vi "On Message.vi"(8 "error in (no error)":errorcluster, 10 "Actor in":refnum<class "Actor.lvclass">, 11 "Client Connection Handler Msg in":refnum<class "Client Connection Handler Msg.lvclass">) -> (0 "error out":errorcluster, 2 "Actor out":refnum<class "Actor.lvclass">, 3 "Client Connection Handler Msg out":refnum<class "Client Connection Handler Msg.lvclass">)   [LabVIEW 2021, in "Echo Broadcast Without Server Manager.lvlib" / "Client Connection Handler Msg.lvclass"]
uses:
  Client Connection Handler Msg.lvclass
  C:/Projects/WebSocket-Actor/WebSocket Actor/Abstract Messages/WebSocket Connection Handler Msg/WebSocket Connection Handler Msg.lvclass
  <vilib>/ActorFramework/Actor/Actor.lvclass
  WS Client/WS Client.lvclass
  C:/Program Files/National Instruments/LabVIEW 2021/vi.lib/ActorFramework/Actor/Actor.lvclass
  WebSocket Actor/Abstract Messages/WebSocket Connection Handler Msg/WebSocket Connection Handler Msg.lvclass/WebSocket Connection Handler Msg.ctl
  WebSocket Actor/Abstract Messages/WebSocket Connection Handler Msg/properties/Read Data.vi
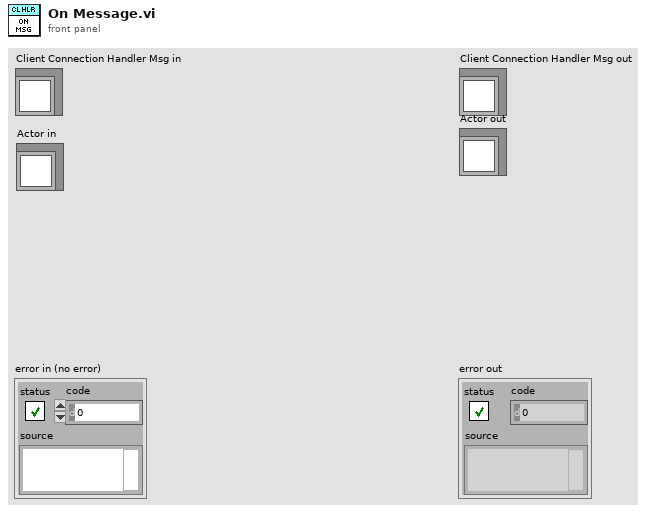
[diagram p1: front panel]
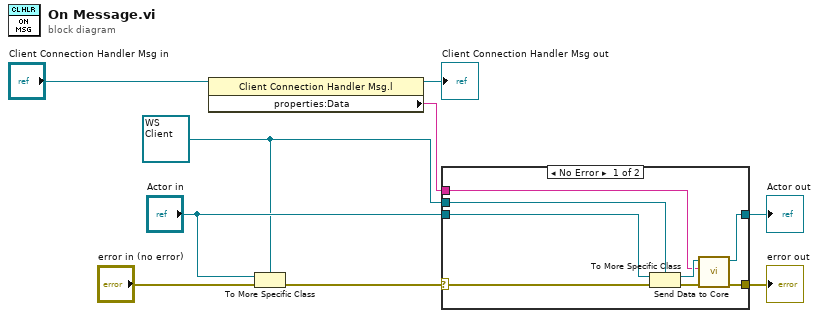
[diagram p0: block diagram]
diagram:
  w3 = refnum<class "WS Client.lvclass"> refnum ("WS Full LabVIEW Test.lvlib:WS Test Client.lvclass")
  n1 = property class="Client Connection Handler Msg.l"(reference="Client Connection Handler Msg in") -> (reference out=→"Client Connection Handler Msg out":refnum<class "Client Connection Handler Msg.lvclass">, "properties:Data"=w2:string)  [unwired: 1 in, 1 out]
  n2 = To More Specific Class(target class=w3, reference="Actor in", error in="error in (no error)") -> (error out=w9:errorcluster)  [unwired: 1 out]
  n3 = case shown="No Error" w9 {
    selector: w9 -> [w16 w18]
    tunnel: "Actor in" -> [w17 w19]
    tunnel: [w14 w18] -> w6
    tunnel: [w13 w19] -> w7
    tunnel: w3 -> [w11 _]
    tunnel: w2 -> [w10 _]
    frame No Error {
      n4 = To More Specific Class(target class=w11, reference=w17, error in=w16) -> (specific class reference=w12:refnum<class "WS Client.lvclass">, error out=w15:errorcluster)
      n5 = call "Send Data to Core.vi"("error in (no error)"=w15, "Data"=w10, "WS Test Client in"=w12) -> ("error out"=w14:errorcluster, "WS Test Client out"=w13:refnum<class "WS Client.lvclass">)  [unwired: 7 in]
    }
    frame Error {
    }
  }
  "error out" <- w6
  "Actor out" <- w7
